vi "gfitsio-open-create-replace-table.vi"(4 "table type (binary)":T1=2 items=["ANY_HDU"=-1, "IMAGE_HDU"=0, "ASCII_TBL"=1, "BINARY_TBL"=2], 5 "prompt (\"Select an HDU\")":string="Select an HDU", 6 "advisory dialog? (display:T)":bool=TRUE, 7 "hdu name (dialog if empty)":string, 8 "error in (no error)":errorcluster, 9 "function (open or create)":T3(ring)=enum."open or create", 11 "gfits refnum":T2) -> (0 "error out":errorcluster, 2 "hdu name out":string, 3 "dup gfits refnum":T2)   [LabVIEW 2011, in "gfitsio.lvlib"]
doc: "Opens an existing FITS table HDU, creates a new FITS table HDU, or replaces an existing FITS table HDU, programmatically or interactively using a dialog box. You can optionally specify a dialog prompt."
uses:
  gfitsio.lvlib
  gfitsio-refnum.ctl
  cfitsio-hdutypes.ctl
  gfitsio-error-codes.ctl
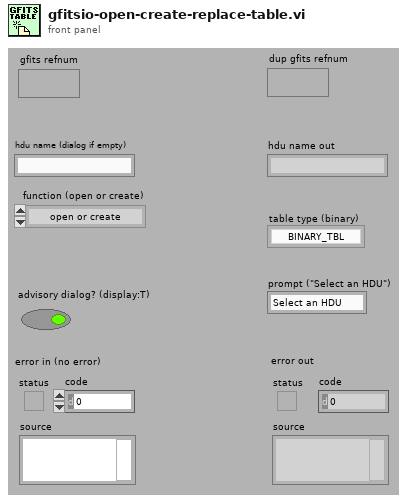
[diagram p1: front panel]
types:
  T1 = typedef "gfitsio.lvlib/cfitsio-hdutypes.ctl" = i32
  T2 = typedef "gfitsio.lvlib/gfitsio-refnum.ctl" = refnum<k1>
  T3 = enum16{"open", "open or create", "create", "create or replace"}
  T4 = typedef "gfitsio.lvlib/gfitsio-error-codes.ctl" = i32
  T5 = enum16{"Error", "Ok", "Cancel", "Abort", "Retry", "Ignore", "Yes", "No", "Close", "Help", "Disabled"}
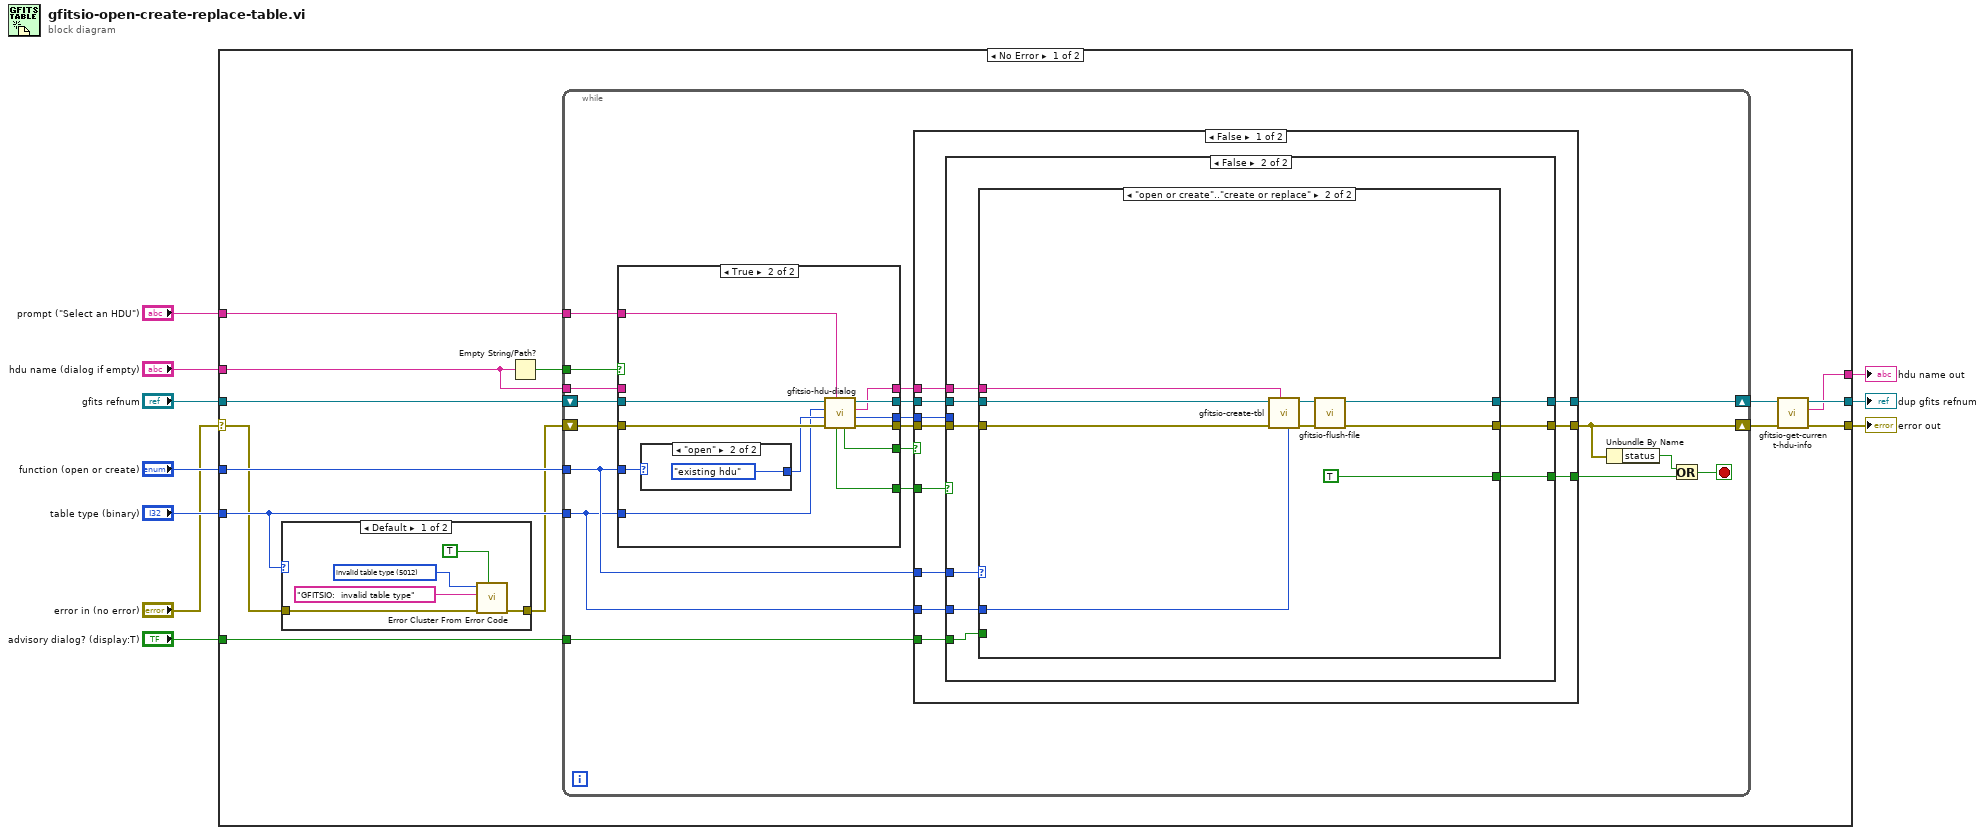
[diagram p0: block diagram]
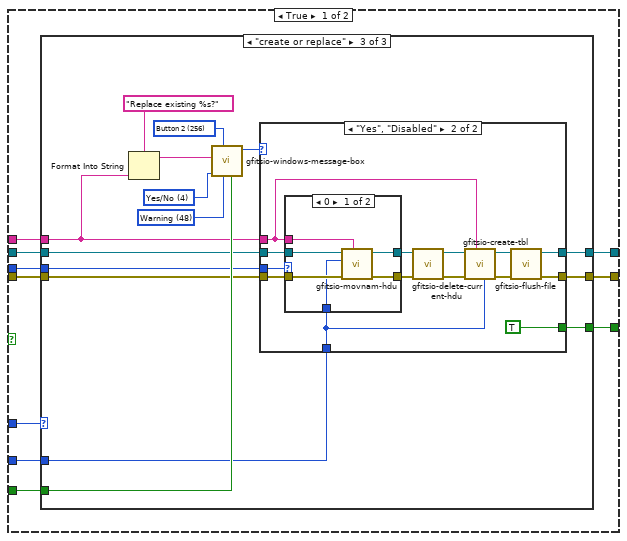
[diagram p3: hidden frame]
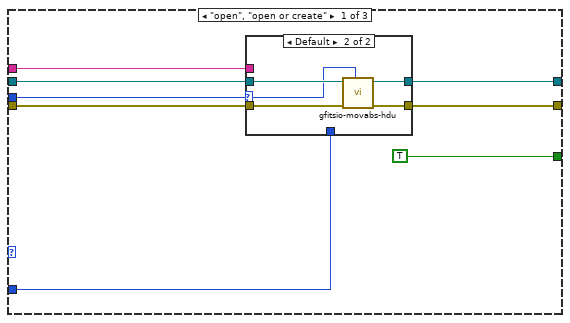
[diagram p4: hidden frame]
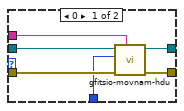
[diagram p5: hidden frame]
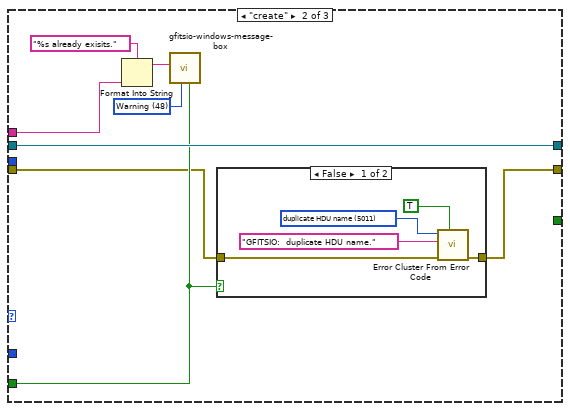
[diagram p6: hidden frame]
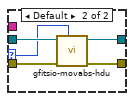
[diagram p9: hidden frame]
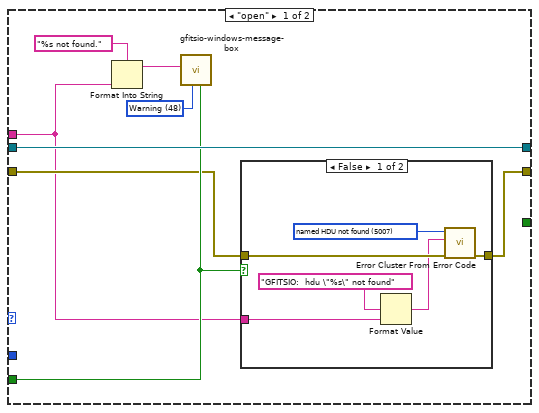
[diagram p10: hidden frame]
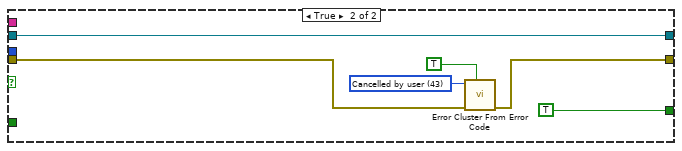
[diagram p12: hidden frame]
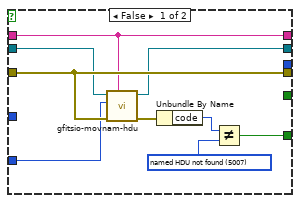
[diagram p13: hidden frame]
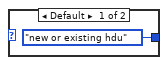
[diagram p14: hidden frame]
diagram:
  n1 = case shown="No Error" "error in (no error)" {
    selector: "error in (no error)" -> [w11 w208]
    tunnel: "advisory dialog? (display:T)" -> [w23 _]
    tunnel: "function (open or create)" -> [w22 _]
    tunnel: "prompt (\"Select an HDU\")" -> [w21 _]
    tunnel: "hdu name (dialog if empty)" -> [w20 _]
    tunnel: "gfits refnum" -> [w19 w209]
    tunnel: [w16 w208] -> w5
    tunnel: [w15 w209] -> w4
    tunnel: [w14 _] -> w3
    tunnel: "table type (binary)" -> [w13 _]
    frame No Error {
      n2 = case shown="Default" w13 {
        tunnel: w11 -> [w29 w30]
        tunnel: [w28 w30] -> w12
        frame Default {
          w25 = T4 5012 items=["no error"=0, "dimensionality conflict"=5001, "fpixel out of image bounds"=5002, "lpixel out of image bounds"=5003, "increment size larger than image"=5004, "increment must be greater than zero"=5005, "fpixel must specify lower left corner"=5006, "named HDU not found"=5007, "specified row is past the end of the table"=5008, "wrong number of elements for column"=5009, "column is not scalar"=5010, "duplicate HDU name"=5011, "invalid table type"=5012] ("Ring")
          n3 = call <vilib>:"Error Cluster From Error Code.vi"("show call chain? (False)"=TRUE, "error in (no error)"=w29, "error message (\"\")"="GFITSIO:  invalid table type" ("error message (\"\")"), "error code (0)"=w25) -> ("error out"=w28:errorcluster)  [unwired: 5 in]
        }
        frame 1, 2 {
        }
      }
      n4 = Empty String/Path?(string/path=w20) -> (empty?=w24:bool)
      n5 = while {
        tunnel: w13 -> [w32]
        tunnel: w22 -> [w33]
        tunnel: w24 -> [w47]
        shift-right: [w42] -> w17
        shift-left: w12 -> [w49]
        shift-right: [w45] -> w18
        shift-left: w19 -> [w48]
        tunnel: w20 -> [w37]
        tunnel: w21 -> [w34]
        tunnel: w23 -> [w31]
        stop <- w39 stop-if-true
        n6 = case shown="True" w47 {
          tunnel: [w193 w205] -> w44
          tunnel: [w191 w204] -> w46
          tunnel: w49 -> [w193 w203]
          tunnel: w48 -> [w192 w202]
          tunnel: w32 -> [w187 w194]
          tunnel: w33 -> [_ w201]
          tunnel: [_ w200] -> w43
          tunnel: [w188 w199] -> w38
          tunnel: w37 -> [w186 _]
          tunnel: [w186 w198] -> w36
          tunnel: [_ w197] -> w35
          tunnel: w34 -> [_ w196]
          frame False {
            w185 = T4 5007 items=["no error"=0, "dimensionality conflict"=5001, "fpixel out of image bounds"=5002, "lpixel out of image bounds"=5003, "increment size larger than image"=5004, "increment must be greater than zero"=5005, "fpixel must specify lower left corner"=5006, "named HDU not found"=5007, "specified row is past the end of the table"=5008, "wrong number of elements for column"=5009, "column is not scalar"=5010, "duplicate HDU name"=5011, "invalid table type"=5012] ("Ring")
            n7 = call "gfitsio-movnam-hdu.vi"("extname"=w186, "error in (no error)"=w193, "hdutype (ANY_HDU)"=w187, "gfits refnum"=w192) -> ("error out"=w190:errorcluster, "dup gfits refnum"=w191:T2)  [unwired: 6 in]
            n8 = Unbundle By Name(w190) -> ("code"=w189:i32)
            n9 = Not Equal?(x=w189, y=w185) -> (x != y?=w188:bool)
          }
          frame True {
            n10 = case shown="\"open\"" w201 {
              tunnel: [enum32{"existing hdu", "new or existing hdu"}."new or existing hdu" ("select mode (new or existing)") enum32{"existing hdu", "new or existing hdu"}."existing hdu" ("select mode (new or existing)")] -> w195
              frame Default {
              }
              frame "open" {
              }
            }
            n11 = call "gfitsio-hdu-dialog.vi"("prompt (\"Select an HDU\")"=w196, "error in (no error)"=w203, "select mode (new or existing)"=w195, "hdu type (ANY_HDU)"=w194, "gfits refnum"=w202) -> ("error out"=w205:errorcluster, "hdu number (0 if cancelled)"=w197:i32, "hdu name (\"\" if cancelled)"=w198:string, "dup gfits refnum"=w204:T2, "cancelled"=w200:bool, "exists"=w199:bool)  [unwired: 1 in]
          }
        }
        n12 = case shown="False" w43 {
          tunnel: w46 -> [w60 w184]
          tunnel: [w57 w184] -> w45
          tunnel: w44 -> [w59 w180]
          tunnel: [w58 w179] -> w42
          tunnel: [w50 TRUE] -> w40
          tunnel: w38 -> [w56 _]
          tunnel: w36 -> [w53 _]
          tunnel: w35 -> [w52 _]
          tunnel: w33 -> [w55 _]
          tunnel: w32 -> [w54 _]
          tunnel: w31 -> [w51 _]
          frame False {
            n13 = case shown="False" w56 {
              tunnel: w60 -> [w68 w152]
              tunnel: w59 -> [w65 w151]
              tunnel: [w66 w150] -> w58
              tunnel: [w67 w149] -> w57
              tunnel: w55 -> [w70 w154]
              tunnel: w54 -> [w69 w153]
              tunnel: w53 -> [w64 w147]
              tunnel: w52 -> [w63 _]
              tunnel: w51 -> [w62 w148]
              tunnel: [w61 w146] -> w50
              frame True {
                n14 = case shown="\"create or replace\"" w70 {
                  tunnel: w69 -> [w72 _ w104]
                  tunnel: w68 -> [w77 w97 w112]
                  tunnel: [w75 w97 w111] -> w67
                  tunnel: [w76 w90 w109] -> w66
                  tunnel: w65 -> [w78 w91 w110]
                  tunnel: w64 -> [w74 w93 w106]
                  tunnel: w63 -> [w73 _ w105]
                  tunnel: w62 -> [_ w92 w113]
                  tunnel: [TRUE _ w107] -> w61
                  frame "open", "open or create" {
                    n15 = case shown="Default" w73 {
                      selector: w73 -> [_ w85]
                      tunnel: w78 -> [w84 w88]
                      tunnel: w77 -> [w83 w89]
                      tunnel: [w82 w87] -> w76
                      tunnel: [w81 w86] -> w75
                      tunnel: w74 -> [w80 _]
                      tunnel: w72 -> [w79 _]
                      frame 0 {
                        n16 = call "gfitsio-movnam-hdu.vi"("extname"=w80, "error in (no error)"=w84, "hdutype (ANY_HDU)"=w79, "gfits refnum"=w83) -> ("error out"=w82:errorcluster, "dup gfits refnum"=w81:T2)  [unwired: 6 in]
                      }
                      frame Default {
                        n17 = call "gfitsio-movabs-hdu.vi"("hdunum"=w85, "error in (no error)"=w88, "gfits refnum"=w89) -> ("error out"=w87:errorcluster, "dup gfits refnum"=w86:T2)  [unwired: 6 in, 1 out]
                      }
                    }
                  }
                  frame "create" {
                    w94 = u32 48 items=["None"=0, "Warning"=48, "Confirmation"=64, "Question"=32, "Error"=16, "User Icon"=128] ("Icon (None)")
                    n18 = Format Into String(format string="%s already exisits.", w93) -> (resulting string=w95:string)  [unwired: 2 in, 1 out]
                    n19 = call "gfitsio-windows-message-box.vi"("enable dialog?"=w92, "Icon (None)"=w94, "Text"=w95) -> ()  [unwired: 8 in, 1 out]
                    n20 = case shown="False" w92 {
                      tunnel: w91 -> [w102 w103]
                      tunnel: [w101 w103] -> w90
                      frame False {
                        w98 = T4 5011 items=["no error"=0, "dimensionality conflict"=5001, "fpixel out of image bounds"=5002, "lpixel out of image bounds"=5003, "increment size larger than image"=5004, "increment must be greater than zero"=5005, "fpixel must specify lower left corner"=5006, "named HDU not found"=5007, "specified row is past the end of the table"=5008, "wrong number of elements for column"=5009, "column is not scalar"=5010, "duplicate HDU name"=5011, "invalid table type"=5012] ("Ring")
                        n21 = call <vilib>:"Error Cluster From Error Code.vi"("show call chain? (False)"=TRUE, "error in (no error)"=w102, "error message (\"\")"="GFITSIO:  duplicate HDU name." ("error message (\"\")"), "error code (0)"=w98) -> ("error out"=w101:errorcluster)  [unwired: 5 in]
                      }
                      frame True {
                      }
                    }
                  }
                  frame "create or replace" {
                    w115 = u32 256 items=["Button 1"=0, "Button 2"=256, "Button 3"=512, "Button 4"=1024] ("Default (Button 1)")
                    w116 = u32 4 items=["Abort/Retry/Ignore"=2, "OK"=0, "OK/Cancel"=1, "Retry/Cancel"=5, "Yes/No"=4, "Yes/No/Cancel"=3] ("Buttons (OK)")
                    w117 = u32 48 items=["None"=0, "Warning"=48, "Confirmation"=64, "Question"=32, "Error"=16, "User Icon"=128] ("Icon (None)")
                    n22 = Format Into String(format string="Replace existing %s?", w106) -> (resulting string=w114:string)  [unwired: 2 in, 1 out]
                    n23 = call "gfitsio-windows-message-box.vi"("enable dialog?"=w113, "Icon (None)"=w117, "Default (Button 1)"=w115, "Buttons (OK)"=w116, "Text"=w114) -> ("Button Selected"=w108:T5)  [unwired: 6 in]
                    n24 = case shown="\"Yes\", \"Disabled\"" w108 {
                      tunnel: w112 -> [w120 w133]
                      tunnel: [w120 w123] -> w111
                      tunnel: w110 -> [w119 w132]
                      tunnel: [w119 w122] -> w109
                      tunnel: [_ TRUE] -> w107
                      tunnel: w106 -> [_ w126]
                      tunnel: w105 -> [_ w131]
                      tunnel: w104 -> [_ w121]
                      frame "No", Default {
                      }
                      frame "Yes", "Disabled" {
                        n25 = case shown="0" w131 {
                          selector: w131 -> [_ w141]
                          tunnel: w132 -> [w140 w144]
                          tunnel: w133 -> [w139 w145]
                          tunnel: [w138 w143] -> w130
                          tunnel: [w137 w142] -> w129
                          tunnel: w126 -> [w136 _]
                          tunnel: w121 -> [w135 _]
                          frame 0 {
                            n26 = call "gfitsio-movnam-hdu.vi"("extname"=w136, "error in (no error)"=w140, "hdutype (ANY_HDU)"=w135, "gfits refnum"=w139) -> ("error out"=w138:errorcluster, "dup gfits refnum"=w137:T2)  [unwired: 6 in]
                          }
                          frame Default {
                            n27 = call "gfitsio-movabs-hdu.vi"("hdunum"=w141, "error in (no error)"=w144, "gfits refnum"=w145) -> ("error out"=w143:errorcluster, "dup gfits refnum"=w142:T2)  [unwired: 6 in, 1 out]
                          }
                        }
                        n28 = call "gfitsio-delete-current-hdu.vi"("error in (no error)"=w130, "gfits refnum"=w129) -> ("error out"=w127:errorcluster, "dup gfits refnum"=w128:T2)  [unwired: 8 in]
                        n29 = call "gfitsio-create-tbl.vi"("tbltype"=w121, "extname"=w126, "error in (no error)"=w127, "gfits refnum"=w128) -> ("error out"=w125:errorcluster, "dup gfits refnum"=w124:T2)  [unwired: 6 in]
                        n30 = call "gfitsio-flush-file.vi"("error in (no error)"=w125, "gfits refnum"=w124) -> ("error out"=w122:errorcluster, "dup gfits refnum"=w123:T2)  [unwired: 8 in]
                      }
                    }
                  }
                }
              }
              frame False {
                n31 = case shown="\"open or create\"..\"create or replace\"" w154 {
                  tunnel: w153 -> [_ w170]
                  tunnel: w152 -> [w162 w177]
                  tunnel: w151 -> [w157 w178]
                  tunnel: [w156 w172] -> w150
                  tunnel: [w162 w171] -> w149
                  tunnel: w148 -> [w158 _]
                  tunnel: w147 -> [w155 w176]
                  tunnel: [_ TRUE] -> w146
                  frame "open" {
                    w159 = u32 48 items=["None"=0, "Warning"=48, "Confirmation"=64, "Question"=32, "Error"=16, "User Icon"=128] ("Icon (None)")
                    n32 = Format Into String(format string="%s not found.", w155) -> (resulting string=w160:string)  [unwired: 2 in, 1 out]
                    n33 = call "gfitsio-windows-message-box.vi"("enable dialog?"=w158, "Icon (None)"=w159, "Text"=w160) -> ()  [unwired: 8 in, 1 out]
                    n34 = case shown="False" w158 {
                      tunnel: w157 -> [w168 w169]
                      tunnel: [w167 w169] -> w156
                      tunnel: w155 -> [w165 _]
                      frame False {
                        w163 = T4 5007 items=["no error"=0, "dimensionality conflict"=5001, "fpixel out of image bounds"=5002, "lpixel out of image bounds"=5003, "increment size larger than image"=5004, "increment must be greater than zero"=5005, "fpixel must specify lower left corner"=5006, "named HDU not found"=5007, "specified row is past the end of the table"=5008, "wrong number of elements for column"=5009, "column is not scalar"=5010, "duplicate HDU name"=5011, "invalid table type"=5012] ("Ring")
                        n35 = Format Value(format string="GFITSIO:  hdu \"%s\" not found", value (0)=w165) -> (output string=w164:string)  [unwired: 1 in]
                        n36 = call <vilib>:"Error Cluster From Error Code.vi"("error in (no error)"=w168, "error message (\"\")"=w164, "error code (0)"=w163) -> ("error out"=w167:errorcluster)  [unwired: 6 in]
                      }
                      frame True {
                      }
                    }
                  }
                  frame "open or create".."create or replace" {
                    n37 = call "gfitsio-create-tbl.vi"("tbltype"=w170, "extname"=w176, "error in (no error)"=w178, "gfits refnum"=w177) -> ("error out"=w174:errorcluster, "dup gfits refnum"=w173:T2)  [unwired: 6 in]
                    n38 = call "gfitsio-flush-file.vi"("error in (no error)"=w174, "gfits refnum"=w173) -> ("error out"=w172:errorcluster, "dup gfits refnum"=w171:T2)  [unwired: 8 in]
                  }
                }
              }
            }
          }
          frame True {
            w182 = 43 items=["No error", "Argument error", "Memory is full", "Out of zone", "End of file", "File already open", "Generic file I/O error", "File not found", "File permission error", "Disk is full", "Duplicate path", "Too many files open", "System feature not enabled", "Resource file not found", "Cannot add resource", "Resource not found", "Image not found", "Image memory error", "Pen does not exist", "Config type invalid", "Config token not found", "Config parse error", "Config memory error", "Bad external code format", "Bad external code offset", "External code not present", "Null window", "Destroy window error", "Null menu", "Print aborted", "Bad print record", "Print driver error", "Windows error during printing", "Memory error during printing", "Print dialog error", "Generic print error", "Invalid device refnum", "Device not found", "Device parameter error", "Device unit error", "Cannot open device", "Device call aborted", "Generic error", "Cancelled by user", "Object ID too low", "Object ID too high", "Object not in heap", "Unknown heap", "Unknown object (invalid DefProc)", "Unknown object (DefProc not in table)", "Message out of range", "Invalid (null) method", "Unknown message", "Manager call not supported", "Bad address", "Network operation in progress", "Network operation timed out", "Connection is busy", "Network attribute not supported", "Network error", "Address in use", "System out of memory", "Connection aborted", "Connection refused", "Not connected", "Already connected", "Connection closed", "Initialization error (interapplication manager)", "Bad occurrence", "Wait on unbound occurrence handler", "Occurrence queue overflow", "Datalog type conflict", "Unused", "Unrecognized type (interapplication manager)", "Memory corrupt", "Failed to make temporary DLL", "Old CIN version", "Drag socket not found", "Failed to load drop-object", "Failed to register OLE object", "Failed to release OLE object", "Format specifier type mismatch", "Unknown format specifier", "Too few format specifiers", "Too many format specifiers", "Scan failed", "Newer CIN version", "Error converting to variant", "Runtime menu error", "Password tampered", "Variant attribute not found", "Incompatible variant data type", "Event data is not available", "Event Store is not present", "Occurrence is not found", "Event Queue is not created", "Event info is not available in the type library", "Refnum passed is NULL", "Error retrieving Class GUID", "Error retrieving CoClass GUID", "Error retrieving TypeLib GUID.", "Bad built application magic bytes.", "Specific driver is different from the specific driver associated with the Logical Name.", "There is no session opened to the class driver.", "Max Error", "MAX - Error with config objects", "MAX - Error loading configuration", "MAX - Group not supported", "Singlecast connections can not send to multicast addresses.", "Multicast connections can not send to singlecast addresses.", "Specified IP address not in multicast address range.", "Attempt to write to read-only multicast connection.", "Attempt to read from write-only multicast connection.", "The buffer used to receive a datagram was smaller than the datagram itself"]
            n39 = call <vilib>:"Error Cluster From Error Code.vi"("show call chain? (False)"=TRUE, "error in (no error)"=w180, "error code (0)"=w182) -> ("error out"=w179:errorcluster)  [unwired: 6 in]
          }
        }
        n40 = Unbundle By Name(w42) -> ("status"=w41:bool)
        n41 = Or(x=w41, y=w40) -> (x .or. y?=w39:bool)
      }
      n42 = call "gfitsio-get-current-hdu-info.vi"("error in (no error)"=w17, "gfits refnum"=w18) -> ("error out"=w16:errorcluster, "hdu name"=w14:string, "dup gfits refnum"=w15:T2)  [unwired: 5 in, 2 out]
    }
    frame Error {
    }
  }
  "error out" <- w5
  "dup gfits refnum" <- w4
  "hdu name out" <- w3
